vi "Translation3d_GetXYZ.vi"(11 "In Translation3d":T1 {"Z" format="%14.3f"; "Y" format="%14.3f"; "X" format="%14.3f"}) -> (1 "Z":dbl, 2 "Y":dbl, 3 "X":dbl)   [LabVIEW 2019, in "Trajectory_Library.lvlib"]
doc: "Returns the X and Ycomponents of the translation.\n\nParameters\n - IN Translation - This Translation data structure\n\nReturns:\n - X- The X component of the translation.\n - Y- The Y component of the translation."
uses:
  Trajectory_Library.lvlib
  TRANSLATION3D.ctl
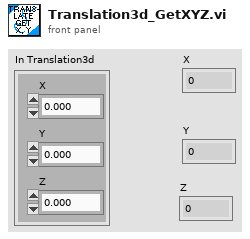
[diagram p1: front panel]
types:
  T1 = typedef "Trajectory_Library.lvlib/TRANSLATION3D.ctl" = cluster{"X":dbl, "Y":dbl, "Z":dbl}
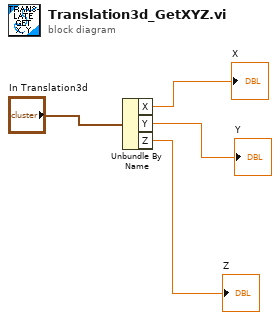
[diagram p0: block diagram]
diagram:
  n1 = Unbundle By Name("In Translation3d") -> ("X"=→"X":dbl, "Y"=→"Y":dbl, "Z"=→"Z":dbl)
